vi "Snake Contains Coordinate.vi"(8 "error in (no error)":errorcluster, 10 "Coordinate":T1, 11 "Snake in":refnum<class "Snake.lvclass">) -> (0 "error out":errorcluster, 2 "In Snake?":bool, 3 "Snake out":refnum<class "Snake.lvclass">)   [LabVIEW 2019, in "Snake.lvclass"]
uses:
  Snake.lvclass
  Coordinate STYP.ctl
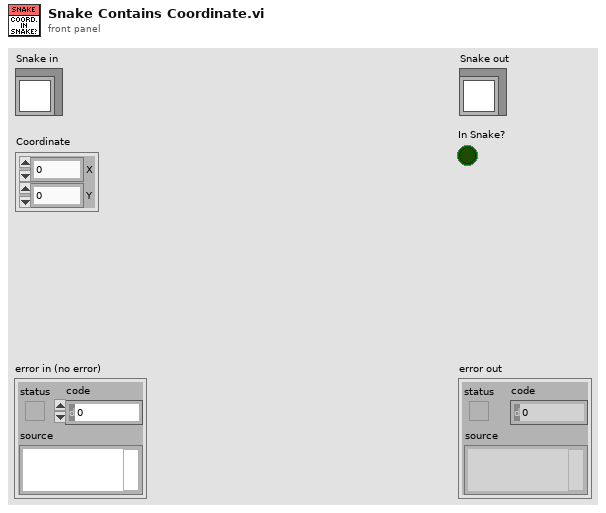
[diagram p1: front panel]
types:
  T1 = typedef "Coordinate STYP.ctl" = cluster{"X":i32, "Y":i32}
  T2 = typedef "Snake.lvclass/Snake Component STYP.ctl" = cluster{"Direction":T3, "Coordinate":T1}
  T3 = typedef "Direction STYP.ctl" = enum16{"Up", "Down", "Left", "Right"}
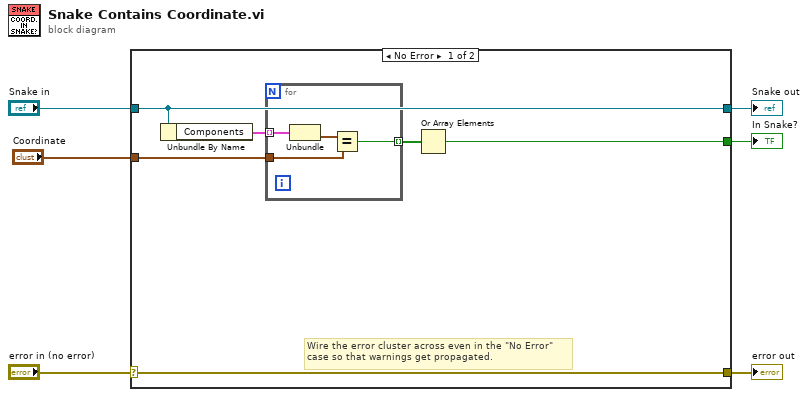
[diagram p0: block diagram]
diagram:
  n1 = case shown="No Error" "error in (no error)" {
    selector: "error in (no error)" -> [w12 w18]
    tunnel: [w12 w18] -> w5
    tunnel: [w11 w17] -> w3
    tunnel: "Snake in" -> [w11 w17]
    tunnel: "Coordinate" -> [w9 _]
    tunnel: [w7 _] -> w1
    frame No Error {
      # "Wire the error cluster across even in the \"No Error\"\ncase so that warnings get propagated."
      n2 = Unbundle By Name(w11) -> ("Components"=w10:T2[])
      n3 = for {
        tunnel: w10 -> [w16] mode=indexing
        tunnel: w9 -> [w14]
        tunnel: [w13] -> w8 mode=indexing
        n4 = Unbundle(w16) -> ("Coordinate"=w15:T1)  [unwired: 1 out]
        n5 = Equal?(x=w15, y=w14) -> (x = y?=w13:bool)
      }
      n6 = Or Array Elements(Boolean array=w8) -> (logical OR=w7:bool)
    }
    frame Error {
    }
  }
  "error out" <- w5
  "Snake out" <- w3
  "In Snake?" <- w1
